vi "NumIntegrate_Func_Ax_Bu_K.vi"(6 "K":T1, 8 "U":T1, 9 "B":T1, 10 "X":T1, 11 "A":T1) -> (0 "Error":bool, 3 "output matrix":T1)   [LabVIEW 2019, in "Trajectory_Library.lvlib"]
doc: "Creates a new LINEAR SYSTEM data cluster with the specified values. \n\n\nInputs: \n - XXX -- XXX.\n\nOutputs:\n - XXX -- XXX."
uses:
  <vilib>/Analysis/Matrix/Datatypes/RealMatrix.ctl
  Trajectory_Library.lvlib
  <vilib>/Analysis/NI_AALBase.lvlib
  <vilib>/Analysis/baseanly.llb/Real A x B.vi
  <vilib>/Analysis/Matrix/NI_Matrix.lvlib
  <vilib>/Analysis/Matrix/Numeric/Add/Add - RM,RM.vi
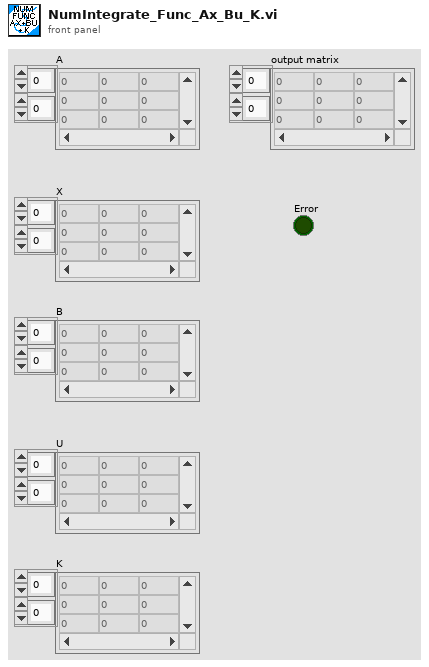
[diagram p1: front panel]
types:
  T1 = typedef "NI_Matrix.lvlib/RealMatrix.ctl" = dbl[][]
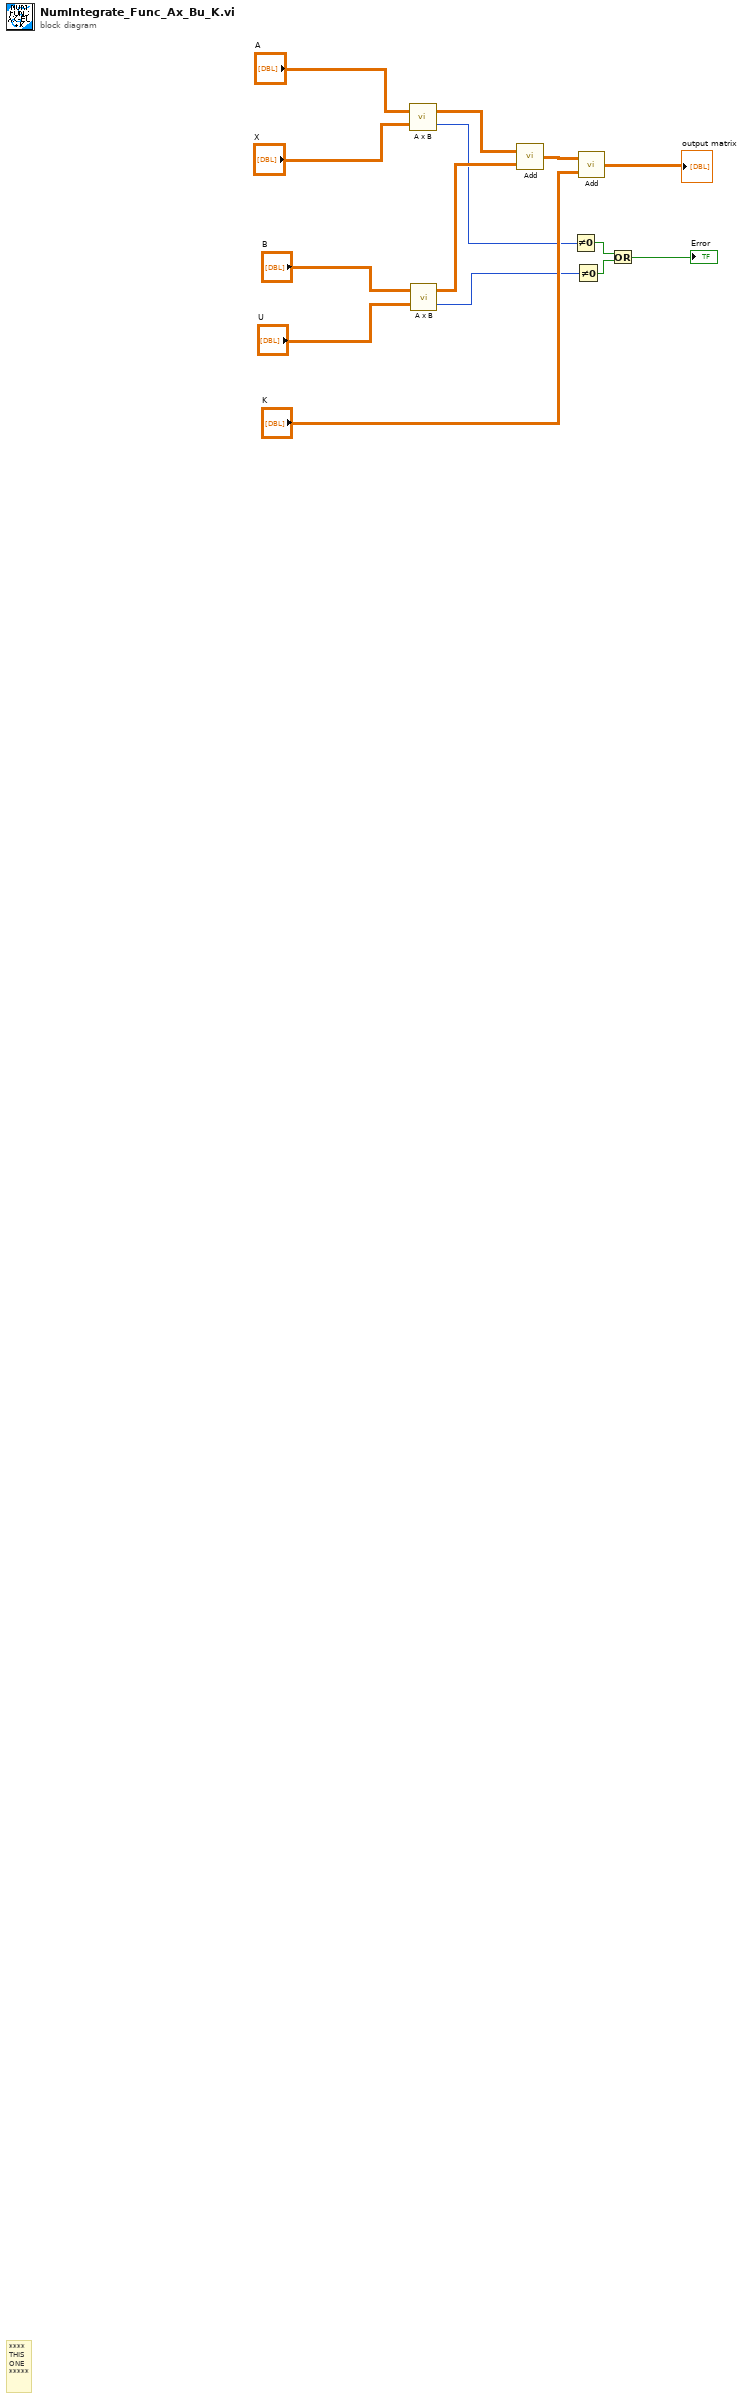
[diagram p0: block diagram]
diagram:
  # "****\nTHIS\nONE\n*****"
  n1 = call-poly <vilib>:"A x B.vi"("B"="X", "A"="A") -> ("error"=w3:i32, "A x B"=w10:T1)
  n2 = call-poly <vilib>:"A x B.vi"("B"="U", "A"="B") -> ("error"=w2:i32, "A x B"=w9:T1)
  n3 = call-poly <vilib>:"Add.vi"("Real Matrix B"=w9, "Real Matrix A"=w10) -> ("A + B"=w8:T1)
  n4 = Not Equal To 0?(x=w3) -> (x != 0?=w5:bool)
  n5 = Not Equal To 0?(x=w2) -> (x != 0?=w4:bool)
  n6 = call-poly <vilib>:"Add.vi"("Real Matrix B"="K", "Real Matrix A"=w8) -> ("A + B"=→"output matrix":T1)
  n7 = Or(x=w5, y=w4) -> (x .or. y?=→"Error":bool)
